vi "Perform Action on Target.vi"(8 "error in":errorcluster, 9 "Input":variant, 10 "Task-Point Ident":string, 11 "Study Actor in":refnum<class "Study Actor.lvclass">) -> (0 "error out":errorcluster, 1 "Output":variant, 2 "Timeout?":bool, 3 "Study Actor out":refnum<class "Study Actor.lvclass">)   [LabVIEW 2024, in "Study Actor.lvlib" / "Study Actor.lvclass"]
uses:
  Study Actor.lvclass
  Study Actor.lvclass/Study Actor.ctl
  <vilib>/ActorFramework/Message Enqueuer/Message Priority.ctl
  HAL/MSS Target Actor/IMSS Target Actor Messages/Perform Action Msg/Perform Action Msg.lvclass/Perform Action Msg.ctl
  HAL/MSS Target Actor/IMSS Target Actor Messages/Perform Action Msg/Perform Action Msg.lvclass
  <vilib>/Utility/error.llb/Error Cluster From Error Code.vi
  Reply-Msg-DataSocket/Reply Msg DataSocket/Send Message and Wait for Response.vi
  <vilib>/ErrorRing/Error Ring.xnode
  <vilib>/ActorFramework/Message Enqueuer/Message Enqueuer.lvclass
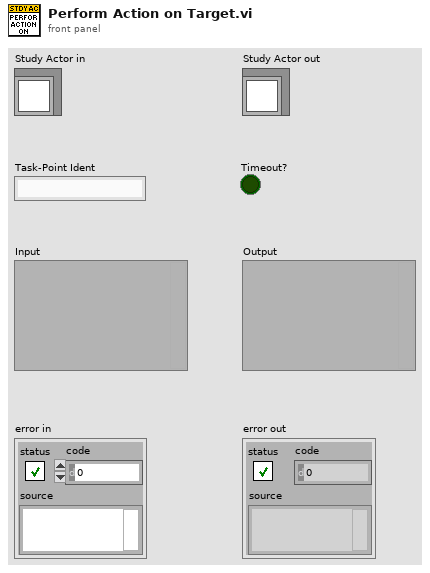
[diagram p1: front panel]
types:
  T1 = typedef "Actor Framework.lvlib/Message Enqueuer.lvclass/Message Priority.ctl" = enum16{"Low", "Normal", "High"}
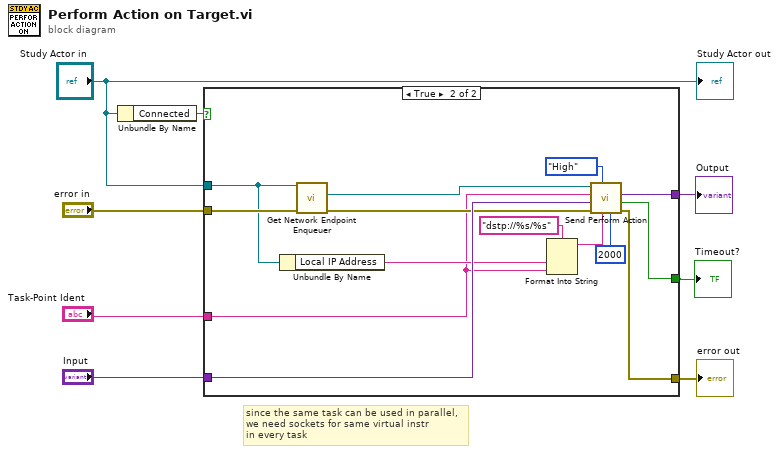
[diagram p0: block diagram]
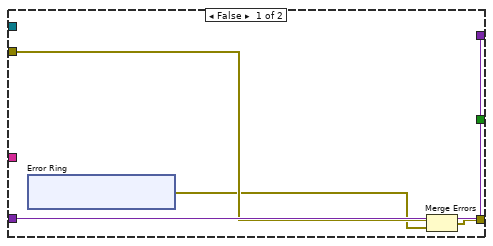
[diagram p2: hidden frame]
diagram:
  # "since the same task can be used in parallel,\nwe need sockets for same virtual instr\nin every task"
  n1 = Unbundle By Name("Study Actor in") -> ("Connected"=w8:bool)
  n2 = case shown="True" w8 {
    tunnel: "Study Actor in" -> [_ w22]
    tunnel: "error in" -> [w11 w31]
    tunnel: [w10 w28] -> w6
    tunnel: "Input" -> [w12 w29]
    tunnel: [w12 w24] -> w4
    tunnel: "Task-Point Ident" -> [_ w18]
    tunnel: [_ w23] -> w2
    frame False {
      n3 = xnode "Error Ring"() -> ("error out"=w9:errorcluster)
      n4 = Merge Errors(w11, w9) -> (w10:errorcluster)
    }
    frame True {
      n5 = Unbundle By Name(w22) -> ("Local IP Address"=w19:string)
      n6 = call "Get Network Endpoint Enqueuer.vi"("error in"=w31, "Study Actor in"=w22) -> ("error out"=w27:errorcluster, "Network Endpoint Enqueuer"=w30:refnum<class "Message Enqueuer.lvclass">)  [unwired: 6 in, 2 out]
      n7 = Format Into String(format string="dstp://%s/%s", w19, w18) -> (resulting string=w21:string)  [unwired: 2 in, 1 out]
      n8 = call "Send Perform Action.vi"("Timeout"=2000, "DataSocket Reply URL"=w21, "Message Priority (Normal)"=Message_Priority."High", "error in (no error)"=w27, "Input"=w29, "Task-Point Ident"=w18, "Message Enqueuer"=w30) -> ("error out"=w28:errorcluster, "Timeout?"=w23:bool, "Reply"=w24:variant)  [unwired: 1 in, 1 out]
    }
  }
  "error out" <- w6
  "Output" <- w4
  "Timeout?" <- w2
  "Study Actor out" <- "Study Actor in"
